vi "Series Recognition.vi"(8 "error in (no error)":errorcluster, 10 "Series Type (0: MXG)":u16(ring) items=["MXG-A", "PSG", "PSG-A", "PSG-C", "PSG-D", "MXG-B", "EXG"], 11 "VISA resource name":refnum<visa-resource-name>) -> (0 "error out":errorcluster, 2 "Is Series Correct":bool, 3 "VISA resource name out":refnum<visa-resource-name>)   [LabVIEW 2014, in "Agilent PSG MXG Series.lvlib"]
doc: "Specifies whether the series is correct."
uses:
  Agilent PSG MXG Series.lvlib
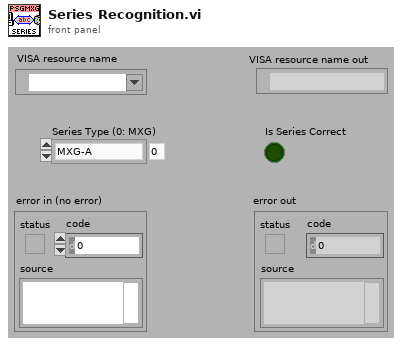
[diagram p1: front panel]
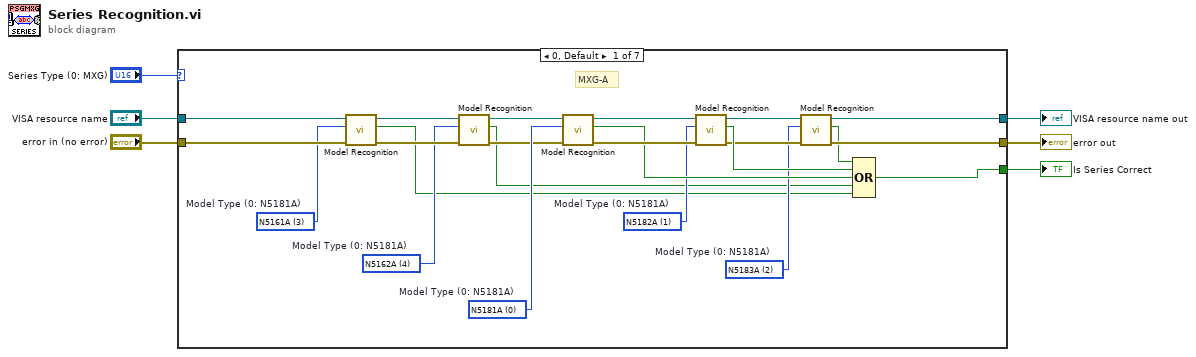
[diagram p0: block diagram]
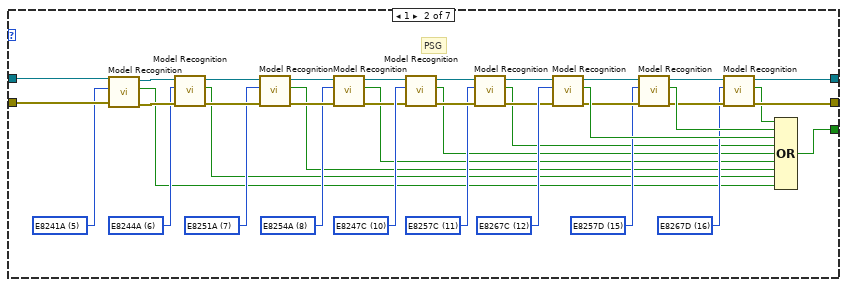
[diagram p2: hidden frame]
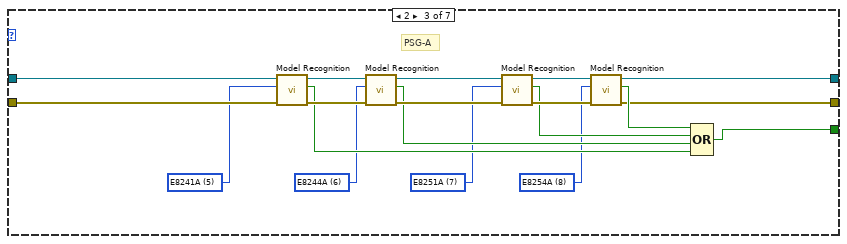
[diagram p3: hidden frame]
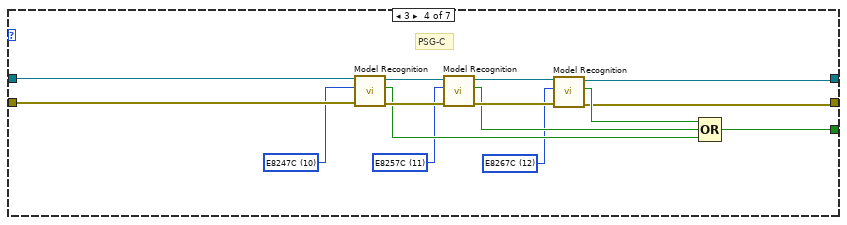
[diagram p4: hidden frame]
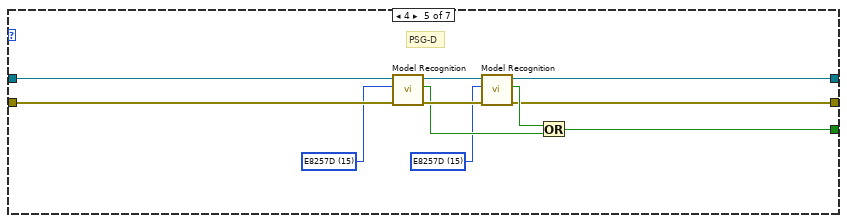
[diagram p5: hidden frame]
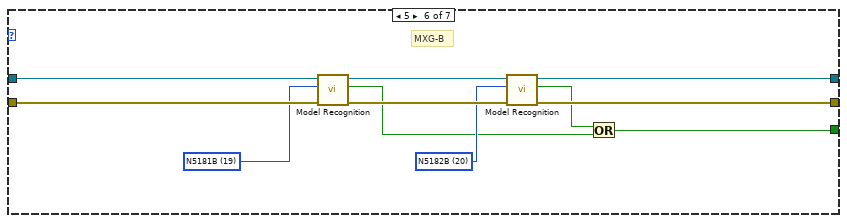
[diagram p6: hidden frame]
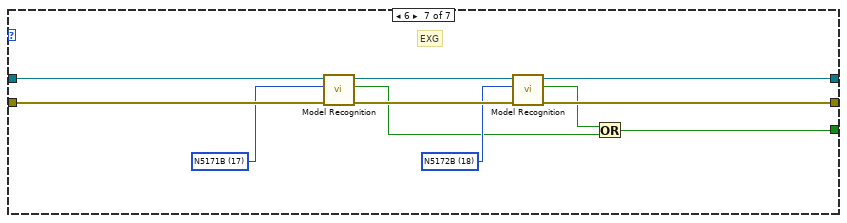
[diagram p7: hidden frame]
diagram:
  n1 = case shown="0, Default" "Series Type (0: MXG)" {
    tunnel: "VISA resource name" -> [w14 w55 w85 w100 w109 w124 w135]
    tunnel: "error in (no error)" -> [w11 w48 w84 w93 w108 w123 w134]
    tunnel: [w25 w59 w75 w94 w107 w114 w125] -> w3
    tunnel: [w20 w62 w74 w92 w106 w121 w132] -> w2
    tunnel: [w19 w61 w73 w91 w105 w119 w130] -> w1
    frame 0, Default {
      w9 = u16 3 items=["N5181A"=0, "N5182A"=1, "N5183A"=2, "N5161A"=3, "N5162A"=4, "E8241A"=5, "E8244A"=6, "E8251A"=7, "E8254A"=8, "E8247C"=10, "E8257C"=11, "E8267C"=12, "E8257D"=15, "E8267D"=16, "N5171B"=17, "N5172B"=18, "N5181B"=19, "N5182B"=20]  # Model Type (0: N5181A)
      w10 = u16 4 items=["N5181A"=0, "N5182A"=1, "N5183A"=2, "N5161A"=3, "N5162A"=4, "E8241A"=5, "E8244A"=6, "E8251A"=7, "E8254A"=8, "E8247C"=10, "E8257C"=11, "E8267C"=12, "E8257D"=15, "E8267D"=16, "N5171B"=17, "N5172B"=18, "N5181B"=19, "N5182B"=20]  # Model Type (0: N5181A)
      w18 = u16 2 items=["N5181A"=0, "N5182A"=1, "N5183A"=2, "E8241A"=5, "E8244A"=6, "E8251A"=7, "E8254A"=8, "E8247C"=10, "E8257C"=11, "E8267C"=12, "E8257D"=15, "E8267D"=16]  # Model Type (0: N5181A)
      w23 = u16 1 items=["N5181A"=0, "N5182A"=1, "E8241A"=5, "E8244A"=6, "E8251A"=7, "E8254A"=8, "E8247C"=10, "E8257C"=11, "E8267C"=12, "E8257D"=15, "E8267D"=16]  # Model Type (0: N5181A)
      w24 = u16 0 items=["N5181A"=0, "N5182A"=1, "E8241A"=5, "E8244A"=6, "E8251A"=7, "E8254A"=8, "E8247C"=10, "E8257C"=11, "E8267C"=12, "E8257D"=15, "E8267D"=16]  # Model Type (0: N5181A)
      # "MXG-A"
      n2 = call "Model Recognition.vi"("error in (no error)"=w11, "Model Type (0: N5181A)"=w9, "VISA resource name"=w14) -> ("error out"=w12:errorcluster, "Is Model Correct"=w7:bool, "VISA resource name out"=w13:refnum<visa-resource-name>)  [unwired: 1 in, 5 out]
      n3 = call "Model Recognition.vi"("error in (no error)"=w12, "Model Type (0: N5181A)"=w10, "VISA resource name"=w13) -> ("error out"=w16:errorcluster, "Is Model Correct"=w8:bool, "VISA resource name out"=w15:refnum<visa-resource-name>)  [unwired: 1 in, 5 out]
      n4 = call "Model Recognition.vi"("error in (no error)"=w16, "Model Type (0: N5181A)"=w24, "VISA resource name"=w15) -> ("error out"=w28:errorcluster, "Is Model Correct"=w27:bool, "VISA resource name out"=w29:refnum<visa-resource-name>)  [unwired: 1 in, 5 out]
      n5 = call "Model Recognition.vi"("error in (no error)"=w28, "Model Type (0: N5181A)"=w23, "VISA resource name"=w29) -> ("error out"=w21:errorcluster, "Is Model Correct"=w26:bool, "VISA resource name out"=w22:refnum<visa-resource-name>)  [unwired: 1 in, 5 out]
      n6 = call "Model Recognition.vi"("error in (no error)"=w21, "Model Type (0: N5181A)"=w18, "VISA resource name"=w22) -> ("error out"=w19:errorcluster, "Is Model Correct"=w17:bool, "VISA resource name out"=w20:refnum<visa-resource-name>)  [unwired: 1 in, 5 out]
      n7 = Compound Arithmetic op=OR(w17, w26, w27, w8, w7) -> (w25:bool)
    }
    frame 1 {
      w37 = u16 5 items=["N5181A"=0, "N5182A"=1, "N5183A"=2, "N5161A"=3, "N5162A"=4, "E8241A"=5, "E8244A"=6, "E8251A"=7, "E8254A"=8, "E8247C"=10, "E8257C"=11, "E8267C"=12, "E8257D"=15, "E8267D"=16, "N5171B"=17, "N5172B"=18, "N5181B"=19, "N5182B"=20] ("Model Type (0: N5181A)")
      w38 = u16 6 items=["N5181A"=0, "N5182A"=1, "N5183A"=2, "N5161A"=3, "N5162A"=4, "E8241A"=5, "E8244A"=6, "E8251A"=7, "E8254A"=8, "E8247C"=10, "E8257C"=11, "E8267C"=12, "E8257D"=15, "E8267D"=16, "N5171B"=17, "N5172B"=18, "N5181B"=19, "N5182B"=20] ("Model Type (0: N5181A)")
      w39 = u16 7 items=["N5181A"=0, "N5182A"=1, "N5183A"=2, "N5161A"=3, "N5162A"=4, "E8241A"=5, "E8244A"=6, "E8251A"=7, "E8254A"=8, "E8247C"=10, "E8257C"=11, "E8267C"=12, "E8257D"=15, "E8267D"=16, "N5171B"=17, "N5172B"=18, "N5181B"=19, "N5182B"=20] ("Model Type (0: N5181A)")
      w40 = u16 8 items=["N5181A"=0, "N5182A"=1, "N5183A"=2, "N5161A"=3, "N5162A"=4, "E8241A"=5, "E8244A"=6, "E8251A"=7, "E8254A"=8, "E8247C"=10, "E8257C"=11, "E8267C"=12, "E8257D"=15, "E8267D"=16, "N5171B"=17, "N5172B"=18, "N5181B"=19, "N5182B"=20] ("Model Type (0: N5181A)")
      w41 = u16 10 items=["N5181A"=0, "N5182A"=1, "N5183A"=2, "N5161A"=3, "N5162A"=4, "E8241A"=5, "E8244A"=6, "E8251A"=7, "E8254A"=8, "E8247C"=10, "E8257C"=11, "E8267C"=12, "E8257D"=15, "E8267D"=16, "N5171B"=17, "N5172B"=18, "N5181B"=19, "N5182B"=20] ("Model Type (0: N5181A)")
      w42 = u16 11 items=["N5181A"=0, "N5182A"=1, "N5183A"=2, "N5161A"=3, "N5162A"=4, "E8241A"=5, "E8244A"=6, "E8251A"=7, "E8254A"=8, "E8247C"=10, "E8257C"=11, "E8267C"=12, "E8257D"=15, "E8267D"=16, "N5171B"=17, "N5172B"=18, "N5181B"=19, "N5182B"=20] ("Model Type (0: N5181A)")
      w56 = u16 12 items=["N5181A"=0, "N5182A"=1, "N5183A"=2, "N5161A"=3, "N5162A"=4, "E8241A"=5, "E8244A"=6, "E8251A"=7, "E8254A"=8, "E8247C"=10, "E8257C"=11, "E8267C"=12, "E8257D"=15, "E8267D"=16, "N5171B"=17, "N5172B"=18, "N5181B"=19, "N5182B"=20] ("Model Type (0: N5181A)")
      w57 = u16 15 items=["N5181A"=0, "N5182A"=1, "N5183A"=2, "N5161A"=3, "N5162A"=4, "E8241A"=5, "E8244A"=6, "E8251A"=7, "E8254A"=8, "E8247C"=10, "E8257C"=11, "E8267C"=12, "E8257D"=15, "E8267D"=16, "N5171B"=17, "N5172B"=18, "N5181B"=19, "N5182B"=20] ("Model Type (0: N5181A)")
      w58 = u16 16 items=["N5181A"=0, "N5182A"=1, "N5183A"=2, "N5161A"=3, "N5162A"=4, "E8241A"=5, "E8244A"=6, "E8251A"=7, "E8254A"=8, "E8247C"=10, "E8257C"=11, "E8267C"=12, "E8257D"=15, "E8267D"=16, "N5171B"=17, "N5172B"=18, "N5181B"=19, "N5182B"=20] ("Model Type (0: N5181A)")
      # "PSG"
      n8 = call "Model Recognition.vi"("error in (no error)"=w48, "Model Type (0: N5181A)"=w37, "VISA resource name"=w55) -> ("error out"=w47:errorcluster, "Is Model Correct"=w30:bool, "VISA resource name out"=w54:refnum<visa-resource-name>)  [unwired: 1 in, 5 out]
      n9 = call "Model Recognition.vi"("error in (no error)"=w47, "Model Type (0: N5181A)"=w38, "VISA resource name"=w54) -> ("error out"=w46:errorcluster, "Is Model Correct"=w31:bool, "VISA resource name out"=w53:refnum<visa-resource-name>)  [unwired: 1 in, 5 out]
      n10 = call "Model Recognition.vi"("error in (no error)"=w46, "Model Type (0: N5181A)"=w39, "VISA resource name"=w53) -> ("error out"=w45:errorcluster, "Is Model Correct"=w32:bool, "VISA resource name out"=w52:refnum<visa-resource-name>)  [unwired: 1 in, 5 out]
      n11 = call "Model Recognition.vi"("error in (no error)"=w45, "Model Type (0: N5181A)"=w40, "VISA resource name"=w52) -> ("error out"=w35:errorcluster, "Is Model Correct"=w33:bool, "VISA resource name out"=w51:refnum<visa-resource-name>)  [unwired: 1 in, 5 out]
      n12 = call "Model Recognition.vi"("error in (no error)"=w35, "Model Type (0: N5181A)"=w41, "VISA resource name"=w51) -> ("error out"=w44:errorcluster, "Is Model Correct"=w34:bool, "VISA resource name out"=w50:refnum<visa-resource-name>)  [unwired: 1 in, 5 out]
      n13 = call "Model Recognition.vi"("error in (no error)"=w44, "Model Type (0: N5181A)"=w42, "VISA resource name"=w50) -> ("error out"=w43:errorcluster, "Is Model Correct"=w36:bool, "VISA resource name out"=w49:refnum<visa-resource-name>)  [unwired: 1 in, 5 out]
      n14 = call "Model Recognition.vi"("error in (no error)"=w43, "Model Type (0: N5181A)"=w56, "VISA resource name"=w49) -> ("error out"=w66:errorcluster, "Is Model Correct"=w67:bool, "VISA resource name out"=w65:refnum<visa-resource-name>)  [unwired: 1 in, 5 out]
      n15 = call "Model Recognition.vi"("error in (no error)"=w66, "Model Type (0: N5181A)"=w57, "VISA resource name"=w65) -> ("error out"=w63:errorcluster, "Is Model Correct"=w68:bool, "VISA resource name out"=w64:refnum<visa-resource-name>)  [unwired: 1 in, 5 out]
      n16 = call "Model Recognition.vi"("error in (no error)"=w63, "Model Type (0: N5181A)"=w58, "VISA resource name"=w64) -> ("error out"=w61:errorcluster, "Is Model Correct"=w60:bool, "VISA resource name out"=w62:refnum<visa-resource-name>)  [unwired: 1 in, 5 out]
      n17 = Compound Arithmetic op=OR(w60, w68, w67, w36, w34, w33, w32, w31, w30) -> (w59:bool)
    }
    frame 2 {
      w69 = u16 8 items=["N5181A"=0, "N5182A"=1, "E8241A"=5, "E8244A"=6, "E8251A"=7, "E8254A"=8, "E8247C"=10, "E8257C"=11, "E8267C"=12, "E8257D"=15, "E8267D"=16] ("Model Type (0: N5181A)")
      w70 = u16 7 items=["N5181A"=0, "N5182A"=1, "E8241A"=5, "E8244A"=6, "E8251A"=7, "E8254A"=8, "E8247C"=10, "E8257C"=11, "E8267C"=12, "E8257D"=15, "E8267D"=16] ("Model Type (0: N5181A)")
      w71 = u16 6 items=["N5181A"=0, "N5182A"=1, "E8241A"=5, "E8244A"=6, "E8251A"=7, "E8254A"=8, "E8247C"=10, "E8257C"=11, "E8267C"=12, "E8257D"=15, "E8267D"=16] ("Model Type (0: N5181A)")
      w72 = u16 5 items=["N5181A"=0, "N5182A"=1, "E8241A"=5, "E8244A"=6, "E8251A"=7, "E8254A"=8, "E8247C"=10, "E8257C"=11, "E8267C"=12, "E8257D"=15, "E8267D"=16] ("Model Type (0: N5181A)")
      # "PSG-A"
      n18 = call "Model Recognition.vi"("error in (no error)"=w84, "Model Type (0: N5181A)"=w72, "VISA resource name"=w85) -> ("error out"=w87:errorcluster, "Is Model Correct"=w79:bool, "VISA resource name out"=w86:refnum<visa-resource-name>)  [unwired: 1 in, 5 out]
      n19 = call "Model Recognition.vi"("error in (no error)"=w87, "Model Type (0: N5181A)"=w71, "VISA resource name"=w86) -> ("error out"=w80:errorcluster, "Is Model Correct"=w78:bool, "VISA resource name out"=w81:refnum<visa-resource-name>)  [unwired: 1 in, 5 out]
      n20 = call "Model Recognition.vi"("error in (no error)"=w80, "Model Type (0: N5181A)"=w70, "VISA resource name"=w81) -> ("error out"=w83:errorcluster, "Is Model Correct"=w77:bool, "VISA resource name out"=w82:refnum<visa-resource-name>)  [unwired: 1 in, 5 out]
      n21 = call "Model Recognition.vi"("error in (no error)"=w83, "Model Type (0: N5181A)"=w69, "VISA resource name"=w82) -> ("error out"=w73:errorcluster, "Is Model Correct"=w76:bool, "VISA resource name out"=w74:refnum<visa-resource-name>)  [unwired: 1 in, 5 out]
      n22 = Compound Arithmetic op=OR(w76, w77, w78, w79) -> (w75:bool)
    }
    frame 3 {
      w88 = u16 12 items=["N5181A"=0, "N5182A"=1, "E8241A"=5, "E8244A"=6, "E8251A"=7, "E8254A"=8, "E8247C"=10, "E8257C"=11, "E8267C"=12, "E8257D"=15, "E8267D"=16] ("Model Type (0: N5181A)")
      w89 = u16 11 items=["N5181A"=0, "N5182A"=1, "E8241A"=5, "E8244A"=6, "E8251A"=7, "E8254A"=8, "E8247C"=10, "E8257C"=11, "E8267C"=12, "E8257D"=15, "E8267D"=16] ("Model Type (0: N5181A)")
      w90 = u16 10 items=["N5181A"=0, "N5182A"=1, "E8241A"=5, "E8244A"=6, "E8251A"=7, "E8254A"=8, "E8247C"=10, "E8257C"=11, "E8267C"=12, "E8257D"=15, "E8267D"=16] ("Model Type (0: N5181A)")
      # "PSG-C"
      n23 = call "Model Recognition.vi"("error in (no error)"=w93, "Model Type (0: N5181A)"=w90, "VISA resource name"=w100) -> ("error out"=w102:errorcluster, "Is Model Correct"=w97:bool, "VISA resource name out"=w101:refnum<visa-resource-name>)  [unwired: 1 in, 5 out]
      n24 = call "Model Recognition.vi"("error in (no error)"=w102, "Model Type (0: N5181A)"=w89, "VISA resource name"=w101) -> ("error out"=w98:errorcluster, "Is Model Correct"=w96:bool, "VISA resource name out"=w99:refnum<visa-resource-name>)  [unwired: 1 in, 5 out]
      n25 = call "Model Recognition.vi"("error in (no error)"=w98, "Model Type (0: N5181A)"=w88, "VISA resource name"=w99) -> ("error out"=w91:errorcluster, "Is Model Correct"=w95:bool, "VISA resource name out"=w92:refnum<visa-resource-name>)  [unwired: 1 in, 5 out]
      n26 = Compound Arithmetic op=OR(w95, w96, w97) -> (w94:bool)
    }
    frame 4 {
      w103 = u16 15 items=["N5181A"=0, "N5182A"=1, "E8241A"=5, "E8244A"=6, "E8251A"=7, "E8254A"=8, "E8247C"=10, "E8257C"=11, "E8267C"=12, "E8257D"=15, "E8267D"=16] ("Model Type (0: N5181A)")
      w104 = u16 15 items=["N5181A"=0, "N5182A"=1, "E8241A"=5, "E8244A"=6, "E8251A"=7, "E8254A"=8, "E8247C"=10, "E8257C"=11, "E8267C"=12, "E8257D"=15, "E8267D"=16] ("Model Type (0: N5181A)")
      # "PSG-D"
      n27 = call "Model Recognition.vi"("error in (no error)"=w108, "Model Type (0: N5181A)"=w104, "VISA resource name"=w109) -> ("error out"=w112:errorcluster, "Is Model Correct"=w111:bool, "VISA resource name out"=w113:refnum<visa-resource-name>)  [unwired: 1 in, 5 out]
      n28 = call "Model Recognition.vi"("error in (no error)"=w112, "Model Type (0: N5181A)"=w103, "VISA resource name"=w113) -> ("error out"=w105:errorcluster, "Is Model Correct"=w110:bool, "VISA resource name out"=w106:refnum<visa-resource-name>)  [unwired: 1 in, 5 out]
      n29 = Or(x=w110, y=w111) -> (x .or. y?=w107:bool)
    }
    frame 5 {
      w117 = u16 19 items=["N5181A"=0, "N5182A"=1, "N5183A"=2, "N5161A"=3, "N5162A"=4, "E8241A"=5, "E8244A"=6, "E8251A"=7, "E8254A"=8, "E8247C"=10, "E8257C"=11, "E8267C"=12, "E8257D"=15, "E8267D"=16, "N5171B"=17, "N5172B"=18, "N5181B"=19, "N5182B"=20] ("Model Type (0: N5181A)")
      w118 = u16 20 items=["N5181A"=0, "N5182A"=1, "N5183A"=2, "N5161A"=3, "N5162A"=4, "E8241A"=5, "E8244A"=6, "E8251A"=7, "E8254A"=8, "E8247C"=10, "E8257C"=11, "E8267C"=12, "E8257D"=15, "E8267D"=16, "N5171B"=17, "N5172B"=18, "N5181B"=19, "N5182B"=20] ("Model Type (0: N5181A)")
      # "MXG-B"
      n30 = call "Model Recognition.vi"("error in (no error)"=w123, "Model Type (0: N5181A)"=w117, "VISA resource name"=w124) -> ("error out"=w120:errorcluster, "Is Model Correct"=w115:bool, "VISA resource name out"=w122:refnum<visa-resource-name>)  [unwired: 1 in, 5 out]
      n31 = call "Model Recognition.vi"("error in (no error)"=w120, "Model Type (0: N5181A)"=w118, "VISA resource name"=w122) -> ("error out"=w119:errorcluster, "Is Model Correct"=w116:bool, "VISA resource name out"=w121:refnum<visa-resource-name>)  [unwired: 1 in, 5 out]
      n32 = Or(x=w116, y=w115) -> (x .or. y?=w114:bool)
    }
    frame 6 {
      w128 = u16 17 items=["N5181A"=0, "N5182A"=1, "N5183A"=2, "N5161A"=3, "N5162A"=4, "E8241A"=5, "E8244A"=6, "E8251A"=7, "E8254A"=8, "E8247C"=10, "E8257C"=11, "E8267C"=12, "E8257D"=15, "E8267D"=16, "N5171B"=17, "N5172B"=18, "N5181B"=19, "N5182B"=20] ("Model Type (0: N5181A)")
      w129 = u16 18 items=["N5181A"=0, "N5182A"=1, "N5183A"=2, "N5161A"=3, "N5162A"=4, "E8241A"=5, "E8244A"=6, "E8251A"=7, "E8254A"=8, "E8247C"=10, "E8257C"=11, "E8267C"=12, "E8257D"=15, "E8267D"=16, "N5171B"=17, "N5172B"=18, "N5181B"=19, "N5182B"=20] ("Model Type (0: N5181A)")
      # "EXG"
      n33 = call "Model Recognition.vi"("error in (no error)"=w134, "Model Type (0: N5181A)"=w128, "VISA resource name"=w135) -> ("error out"=w131:errorcluster, "Is Model Correct"=w126:bool, "VISA resource name out"=w133:refnum<visa-resource-name>)  [unwired: 1 in, 5 out]
      n34 = call "Model Recognition.vi"("error in (no error)"=w131, "Model Type (0: N5181A)"=w129, "VISA resource name"=w133) -> ("error out"=w130:errorcluster, "Is Model Correct"=w127:bool, "VISA resource name out"=w132:refnum<visa-resource-name>)  [unwired: 1 in, 5 out]
      n35 = Or(x=w127, y=w126) -> (x .or. y?=w125:bool)
    }
  }
  "error out" <- w1
  "VISA resource name out" <- w2
  "Is Series Correct" <- w3
